vi "EnQ_Single_Element_String_Variant_TT.vi"(8 "error in (no error)":errorcluster, 9 "Variant":variant, 10 "State":string, 11 "queueIN":refnum<queue>) -> (0 "error out":errorcluster, 3 "queueOUT":refnum<queue>)   [LabVIEW 2018]
panel:
  in  "timeout in ms (-1)":i32
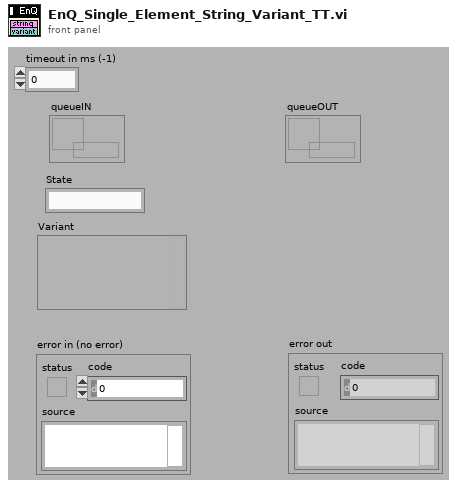
[diagram p1: front panel]
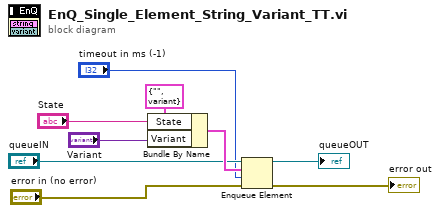
[diagram p0: block diagram]
diagram:
  n1 = Bundle By Name(cluster=cluster{"State":string, "Variant":variant} {"State"="", "Variant"=variant} ("output cluster"), "State"="State", "Variant"="Variant") -> (w6:cluster{"State":string, "Variant":variant})
  n2 = Enqueue Element(queue="queueIN", element=w6, timeout in ms (-1)="timeout in ms (-1)", error in (no error)="error in (no error)") -> (queue out=→"queueOUT":refnum<queue>, error out=→"error out":errorcluster)  [unwired: 1 out]
